vi "Set Previous Row Flags.vi"(9 "Cutoff":i32, 10 "Flag Array":bool[][](array[boolean]), 11 "Match Array":i32[][](array[numeric])) -> (3 "Flag Array Out":bool[][](array[boolean]))   [LabVIEW 2013]
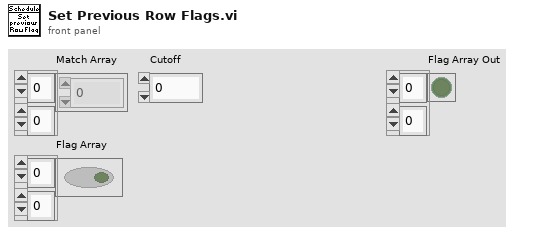
[diagram p1: front panel]
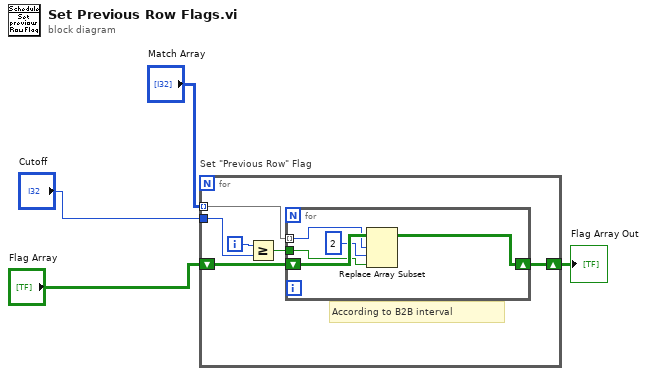
[diagram p0: block diagram]
diagram:
  n1 = for "Set \"Previous Row\" Flag" {
    shift-right: [w5] -> w1
    shift-left: "Flag Array" -> [w7]
    tunnel: "Match Array" -> [w8] mode=indexing
    tunnel: "Cutoff" -> [w10]
    i -> [w9]
    # "According to B2B interval"
    n2 = Greater Or Equal?(x=w9, y=w10) -> (x >= y?=w6:bool)
    n3 = for {
      tunnel: w8 -> [w14] mode=indexing
      tunnel: w6 -> [w12]
      shift-right: [w11] -> w5
      shift-left: w7 -> [w15]
      n4 = Replace Array Subset(array=w15, new element=w12, index (row)=w14, index (col)=2 ("disabled index (col)")) -> (w11:bool[][])
    }
  }
  "Flag Array Out" <- w1
